vi "Write #film appearances.vi"(8 "error in (no error)":errorcluster, 10 "#film appearances":u16, 11 "Bobby Jones in":refnum<class "Bobby Jones.lvclass">) -> (0 "error out":errorcluster, 3 "Bobby Jones out":refnum<class "Bobby Jones.lvclass">)   [LabVIEW 2019, in "Bobby Jones.lvclass"]
uses:
  Bobby Jones.lvclass
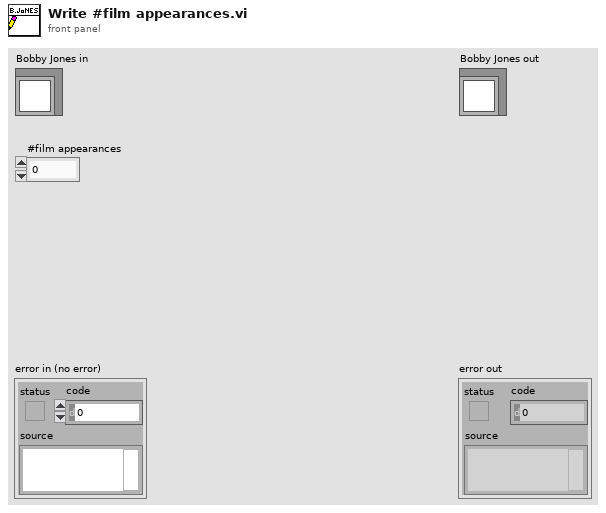
[diagram p1: front panel]
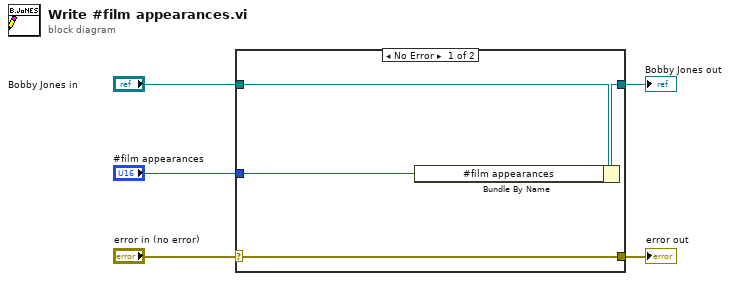
[diagram p0: block diagram]
diagram:
  n1 = case shown="No Error" "error in (no error)" {
    selector: "error in (no error)" -> [w9 w10]
    tunnel: [w9 w10] -> w4
    tunnel: [w7 w11] -> w2
    tunnel: "Bobby Jones in" -> [w8 w11]
    tunnel: "#film appearances" -> [w6 _]
    frame No Error {
      n2 = Bundle By Name(cluster=w8, "#film appearances"=w6) -> (w7:refnum<class "Bobby Jones.lvclass">)
    }
    frame Error {
    }
  }
  "error out" <- w4
  "Bobby Jones out" <- w2
